vi "ech_Ex2Task3_12-13-16.vi"() -> ()   [LabVIEW 2014]
panel:
  out "Avg Value":dbl
  out "Waveform Graph":dynamicdata(graph)
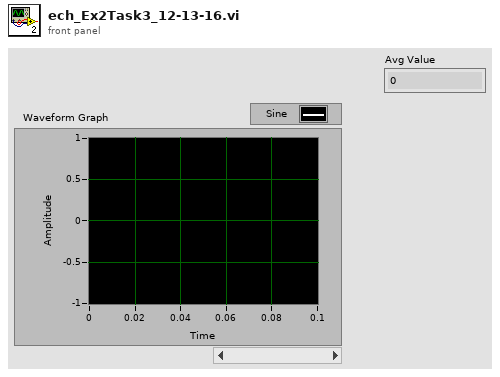
[diagram p1: front panel]
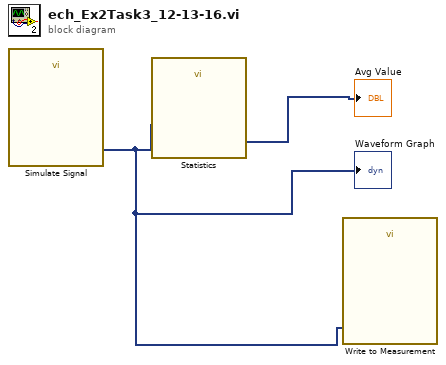
[diagram p0: block diagram]
diagram:
  n1 = call "Simulate Signal"() -> ("Sine"=w1:dynamicdata)  [unwired: 14 in, 1 out]
  "Waveform Graph" <- w1
  n2 = call "Statistics"("Signals"=w1) -> ("Arithmetic Mean"=→"Avg Value":dynamicdata)  [unwired: 25 in, 1 out]
  n3 = call "Write to Measurement"("Signals"=w1) -> ()  [unwired: 16 in, 3 out]
